vi "setCost.vi"(8 "error in (no error)":errorcluster, 10 "cost":dbl, 11 "MintTea in":refnum<class "MintTea.lvclass">) -> (0 "error out":errorcluster, 3 "MintTea out":refnum<class "MintTea.lvclass">)   [LabVIEW 2018, in "MintTea.lvclass"]
uses:
  MintTea.lvclass
  Beverage Class/Beverage.lvclass
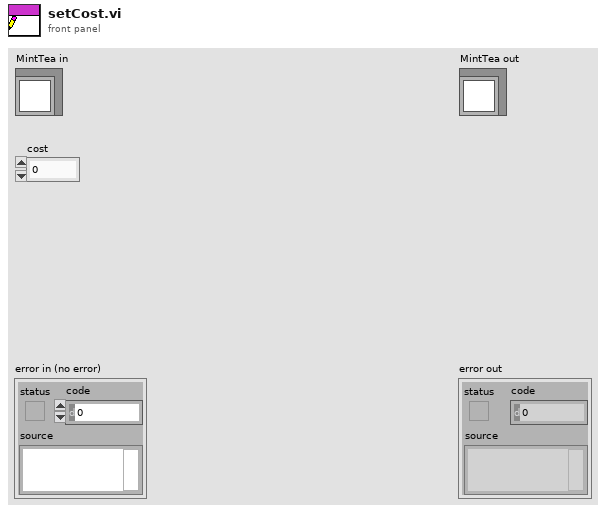
[diagram p1: front panel]
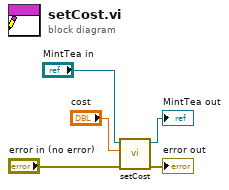
[diagram p0: block diagram]
diagram:
  n1 = call-parent "setCost.vi"("error in (no error)"="error in (no error)", "cost"="cost", "Beverage in"="MintTea in") -> ("error out"=→"error out":errorcluster, "Beverage out"=→"MintTea out":refnum<class "MintTea.lvclass">)  [unwired: 7 in]
